vi "ExtendDevStatus.vi"(7 "error in":errorcluster, 9 "ON/OFF":bool, 10 "VISA resource name in":refnum<visa-resource-name>) -> (0 "error out":errorcluster, 2 "Extend Device Status":T1, 3 "VISA resource name out":refnum<visa-resource-name>)   [LabVIEW 2014]
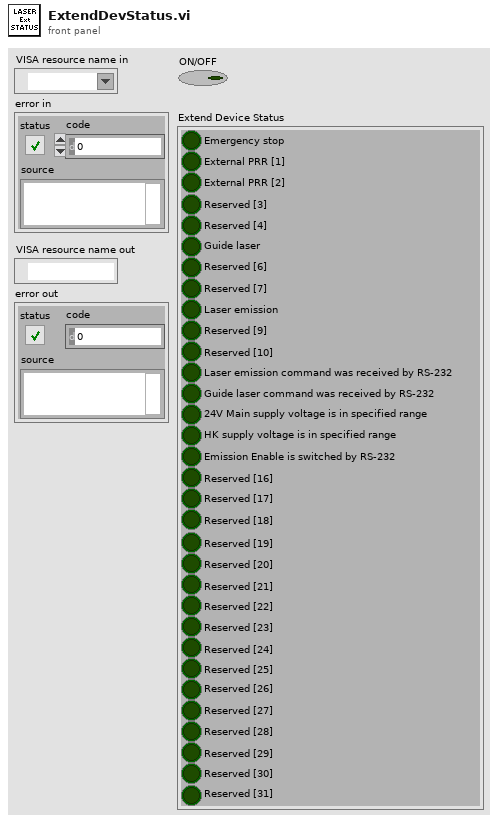
[diagram p1: front panel]
types:
  T1 = cluster{"Emergency stop":bool, "External PRR [1]":bool, "External PRR [2]":bool, "Reserved [3]":bool, "Reserved [4]":bool, "Guide laser":bool, "Reserved [6]":bool, "Reserved [7]":bool, "Laser emission":bool, "Reserved [9]":bool, "Reserved [10]":bool, "Laser emission command was received by RS-232":bool, "Guide laser command was received by RS-232":bool, "24V Main supply voltage is in specified range":bool, "HK supply voltage is in specified range":bool, "Emission Enable is switched by RS-232":bool, "Reserved [16]":bool, "Reserved [17]":bool, "Reserved [18]":bool, "Reserved [19]":bool, "Reserved [20]":bool, "Reserved [21]":bool, "Reserved [22]":bool, "Reserved [23]":bool, "Reserved [24]":bool, "Reserved [25]":bool, "Reserved [26]":bool, "Reserved [27]":bool, "Reserved [28]":bool, "Reserved [29]":bool, "Reserved [30]":bool, "Reserved [31]":bool}
  T2 = cluster{"Boolean array[0]":bool, "Boolean array[1]":bool, "Boolean array[2]":bool, "Boolean array[3]":bool, "Boolean array[4]":bool, "Boolean array[5]":bool, "Boolean array[6]":bool, "Boolean array[7]":bool, "Boolean array[8]":bool, "Boolean array[9]":bool, "Boolean array[10]":bool, "Boolean array[11]":bool, "Boolean array[12]":bool, "Boolean array[13]":bool, "Boolean array[14]":bool, "Boolean array[15]":bool, "Boolean array[16]":bool, "Boolean array[17]":bool, "Boolean array[18]":bool, "Boolean array[19]":bool, "Boolean array[20]":bool, "Boolean array[21]":bool, "Boolean array[22]":bool, "Boolean array[23]":bool, "Boolean array[24]":bool, "Boolean array[25]":bool, "Boolean array[26]":bool, "Boolean array[27]":bool, "Boolean array[28]":bool, "Boolean array[29]":bool, "Boolean array[30]":bool, "Boolean array[31]":bool}
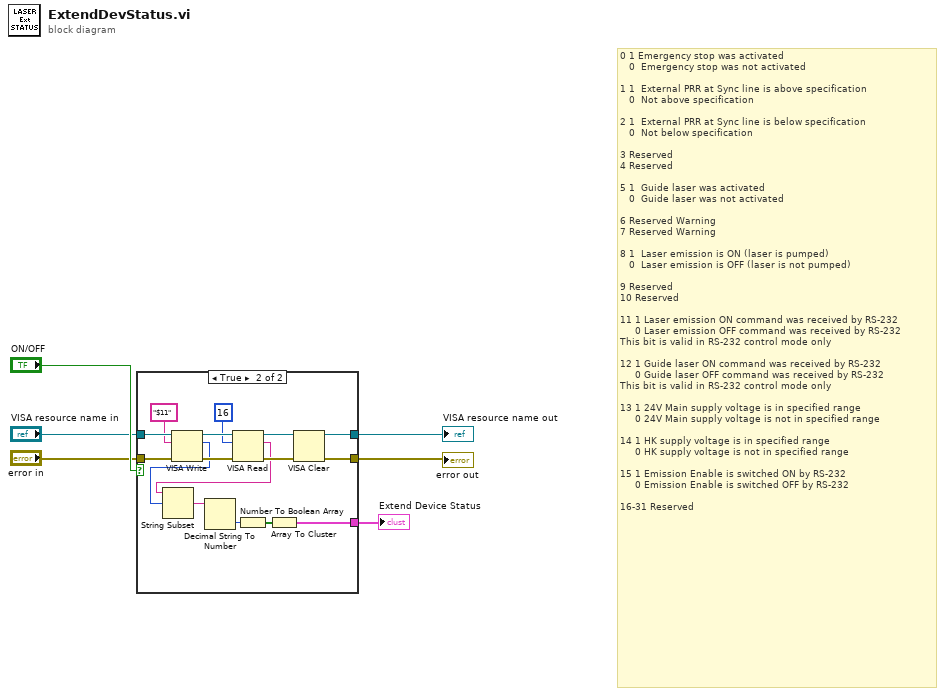
[diagram p0: block diagram]
diagram:
  # "0 1 Emergency stop was activated\n   0  Emergency stop was not activated\n\n1 1  External PRR at Sync line is above specification\n   0  Not above specification\n\n2 1  External PRR at Sync line is below specification\n   0  Not below specification\n\n3 Reserved\n4 Reserved\n\n5 1  Guide laser was activated\n   0  Guide laser was not activated\n\n6 Reserved Warning\n7 Reserved Warning\n\n8 1  Laser emission is ON (laser is pumped)\n   0  Laser emission is OFF (laser is not pumped) \n\n9 Reserved\n10 Reserved\n\n11 1 Laser emission ON command was received by RS-232\n     0 Laser emission OFF command was received by RS-232\nThis bit is valid in RS-232 control mode only\n\n12 1 Guide laser ON command was received by RS-232\n     0 Guide laser OFF command was received by RS-232\nThis bit is valid in RS-232 control mode only\n\n13 1 24V Main supply voltage is in specified range\n     0 24V Main supply voltage is not in specified range\n\n14 1 HK supply voltage is in specified range\n     0 HK supply voltage is not in specified range\n\n15 1 Emission Enable is switched ON by RS-232\n     0 Emission Enable is switched OFF by RS-232\n\n16-31 Reserved"
  n1 = case shown="True" "ON/OFF" {
    tunnel: "VISA resource name in" -> [w8 w22]
    tunnel: "error in" -> [w7 w21]
    tunnel: [w8 w18] -> w3
    tunnel: [w7 w17] -> w2
    tunnel: [_ w10] -> w1
    frame False {
    }
    frame True {
      n2 = VISA Write(VISA resource name=w22, write buffer="$11", error in (no error)=w21) -> (VISA resource name out=w23:refnum<visa-resource-name>, return count=w12:u32, error out=w24:errorcluster)
      n3 = VISA Read(VISA resource name=w23, byte count=u32 16, error in (no error)=w24) -> (VISA resource name out=w20:refnum<visa-resource-name>, read buffer=w13:string, error out=w19:errorcluster)  [unwired: 1 out]
      n4 = String Subset(string=w13, offset (0)=w12) -> (substring=w14:string)  [unwired: 1 in]
      n5 = Decimal String To Number(string=w14) -> (number=w15:i32)  [unwired: 2 in, 1 out]
      n6 = Number To Boolean Array(number=w15) -> (Boolean array=w11:bool[])
      n7 = Array To Cluster(array=w11) -> (cluster=w10:T2)
      n8 = VISA Clear(VISA resource name=w20, error in (no error)=w19) -> (VISA resource name out=w18:refnum<visa-resource-name>, error out=w17:errorcluster)
    }
  }
  "Extend Device Status" <- w1
  "VISA resource name out" <- w3
  "error out" <- w2
